vi "2D Matrix (Demo).vi"() -> ()   [LabVIEW 2014]
uses:
  <vilib>/Analysis/Matrix/Datatypes/RealMatrix.ctl
  <vilib>/Analysis/Matrix/NI_Matrix.lvlib
panel:
  out "2D Matrix":T1
  in  "nRows":i32=1
  in  "nCols":i32
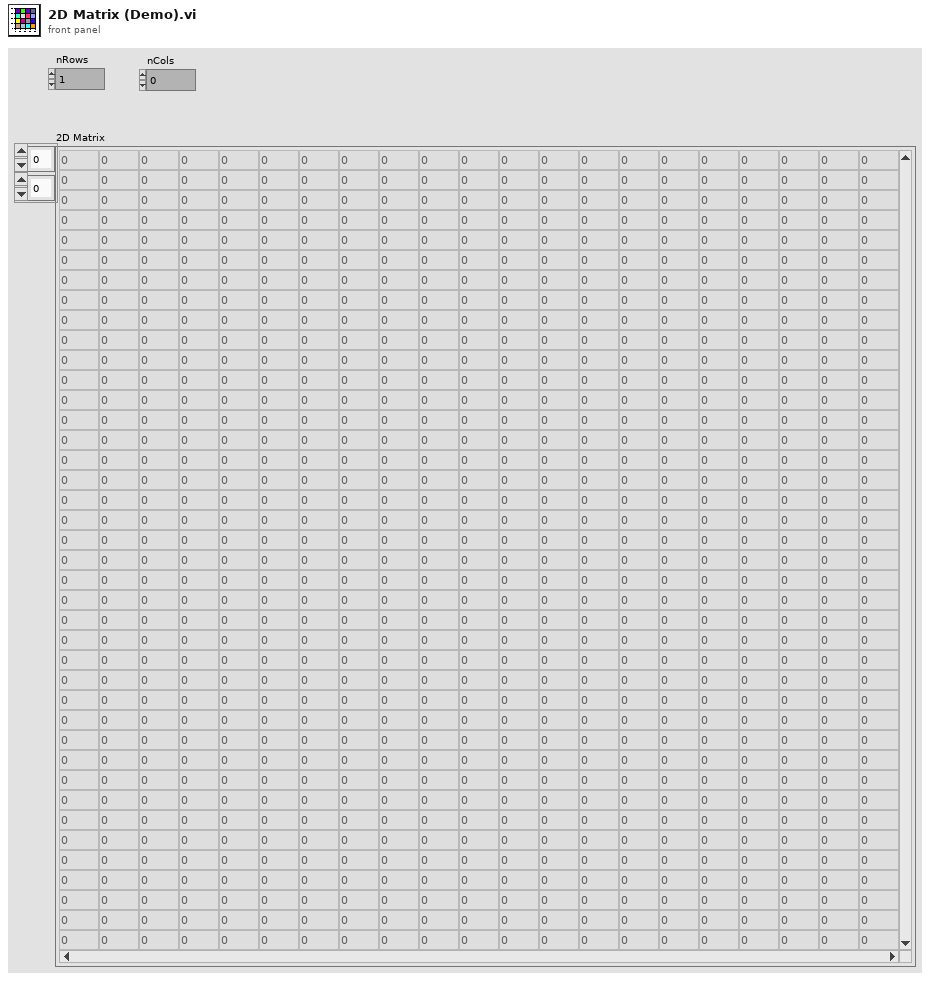
[diagram p1: front panel]
types:
  T1 = typedef "NI_Matrix.lvlib/RealMatrix.ctl" = dbl[][]
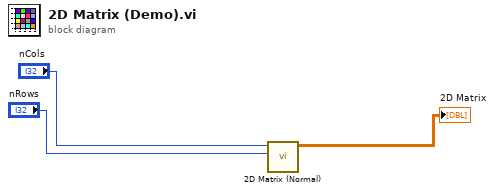
[diagram p0: block diagram]
diagram:
  n1 = call "2D Matrix (Normal).vi"("nRows"="nRows", "nCols"="nCols") -> ("Normal Matrix"=→"2D Matrix":T1)  [unwired: 9 in]
